vi "Tree Get Node (TreePath).vi"(8 "error in (no error)":errorcluster, 10 "Path":refnum<data-value>, 11 "Tree DVR in":refnum<data-value>) -> (0 "error out":errorcluster, 2 "Node out":refnum<data-value>, 3 "Tree DVR out":refnum<data-value>)   [LabVIEW 2012, in "MDSplus.lvlib"]
doc: "Return the TreeNode for the data itemspecified by the passed TreePath instance."
uses:
  <vilib>/MDSplus/Library/MDSplus.lvlib
  <vilib>/MDSplus/Classes/Tree_Class/Tree.lvclass
  <vilib>/MDSplus/Classes/Data_Class/TreeNode_Class/TreeNode.lvclass
  <vilib>/MDSplus/Classes/Data_Class/TreeNode_Class/TreePath_Class/TreePath.lvclass
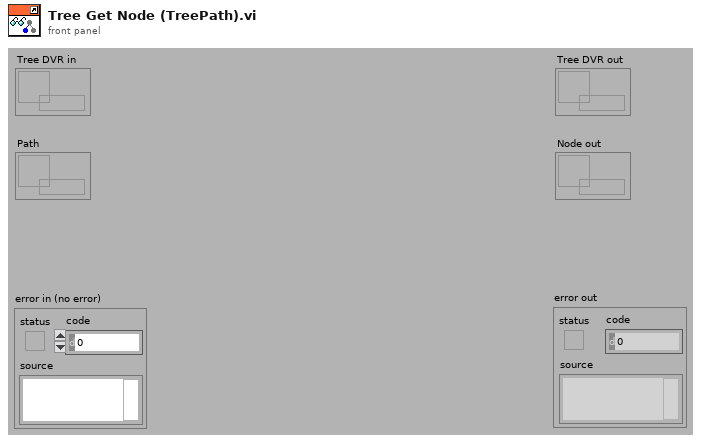
[diagram p1: front panel]
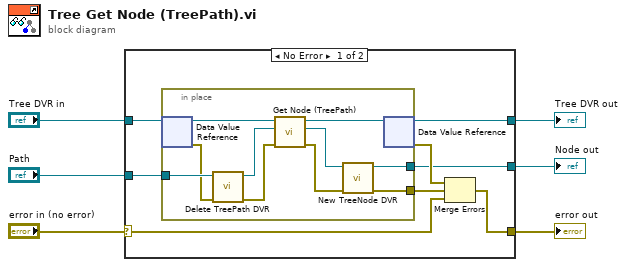
[diagram p0: block diagram]
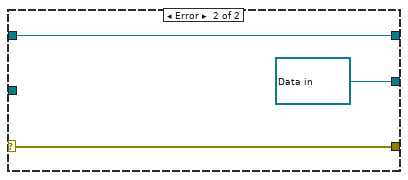
[diagram p2: hidden frame]
diagram:
  n1 = case shown="No Error" "error in (no error)" {
    selector: "error in (no error)" -> [w13 w27]
    tunnel: "Tree DVR in" -> [w14 w26]
    tunnel: [w11 w27] -> w6
    tunnel: [w10 w26] -> w3
    tunnel: [w8 refnum<data-value> refnum ("TreeNode DVR out")] -> w2
    tunnel: "Path" -> [w9 _]
    frame No Error {
      n2 = in-place {
        in-place-border: [w19] -> w7
        in-place-border: w9 -> [w18]
        in-place-border: [w21] -> w8
        n3 = in-place-dvr #1(w14) -> (w24:refnum<class "Tree.lvclass">, w16:errorcluster)
        n4 = call <vilib>:"Delete TreePath DVR.vi"("error in (no error)"=w16, "TreePath DVR in"=w18) -> ("error out"=w15:errorcluster, "TreePath out"=w17:refnum<class "TreePath.lvclass">)  [unwired: 8 in]
        n5 = call-dynamic "Get Node (TreePath).vi"("error in (no error)"=w15, "Path"=w17, "Tree in"=w24) -> ("error out"=w20:errorcluster, "Node out"=w22:refnum<class "TreeNode.lvclass">, "Tree out"=w23:refnum<class "Tree.lvclass">)  [unwired: 6 in]
        n6 = call <vilib>:"New TreeNode DVR.vi"("error in (no error)"=w20, "TreeNode in"=w22) -> ("error out"=w19:errorcluster, "TreeNode DVR out"=w21:refnum<data-value>)  [unwired: 8 in]
        n7 = in-place-dvr #1(w23) -> (w10:refnum<data-value>, w12:errorcluster)
      }
      n8 = Merge Errors(w12, w7, w13) -> (w11:errorcluster)
    }
    frame Error {
    }
  }
  "error out" <- w6
  "Tree DVR out" <- w3
  "Node out" <- w2
